vi "Set Tube State.vi"(4 "State":T1(ring), 5 "valve refs":refnum<vi>[](array[refnum]), 6 "error in":errorcluster, 8 "tube state ref":refnum<vi>, 9 "task in":refnum<k21>) -> (0 "error out":errorcluster, 3 "task out":refnum<k21>)   [LabVIEW 2018]
uses:
  <vilib>/DAQmx/write.llb/DAQmx Write (Digital 1D Bool 1Chan 1Samp).vi
  <vilib>/DAQmx/miscellaneous.llb/DAQmx Fill In Error Info.vi
panel:
  out "Valve Tube Inlet":bool caption="Tube Inlet"
  out "Valve Mix Inlet":bool caption="Mix Inlet"
  out "Valve Mix Outlet":bool caption="Mix Outlet"
  out "Valve Tube Outlet":bool=TRUE caption="Tube Outlet"
  out "Valve Oxidizer":bool caption="Oxidizer"
  out "Valve Fuel":bool caption="Fuel"
  out "Valve Diluent":bool caption="Diluent"
  out "Valve Purge":bool caption="Purge"
  out "Valve Vacuum":bool caption="Vacuum"
  out "Spark":bool
  out "Mix Fan":bool
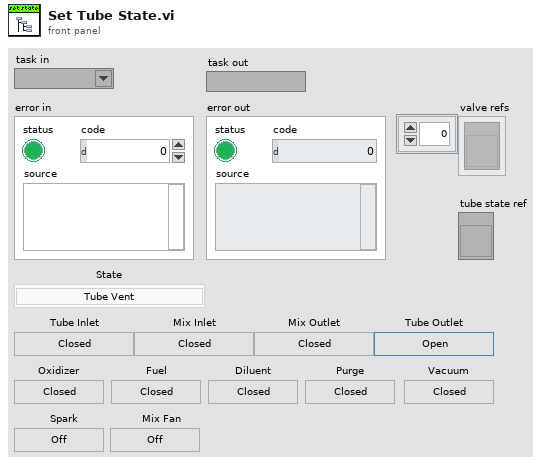
[diagram p1: front panel]
types:
  T1 = enum16{"Tube Vent", "Mix Section Purge", "Tube Purge", "Tube Vacuum", "Diluent Fill", "Oxidizer Fill", "Fuel Fill", "Fill Hold", "Mixing", "Tube Closed", "Ignition", "Manifold Vent"}
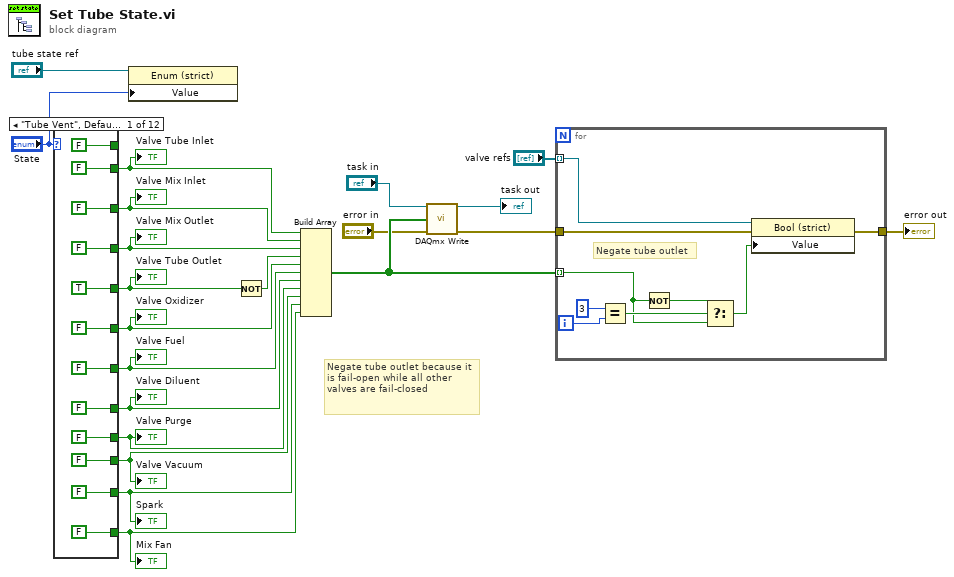
[diagram p0: block diagram]
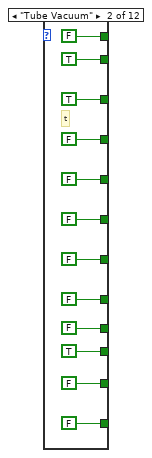
[diagram p2: hidden frame]
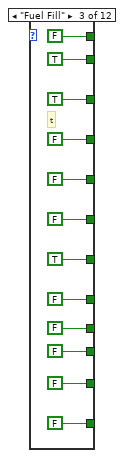
[diagram p3: hidden frame]
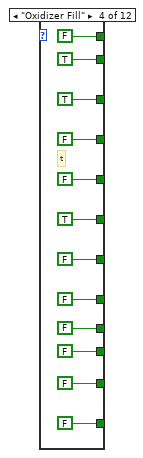
[diagram p4: hidden frame]
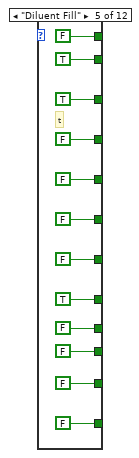
[diagram p5: hidden frame]
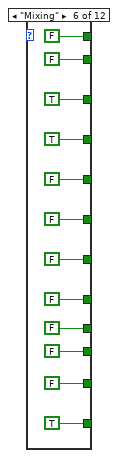
[diagram p6: hidden frame]
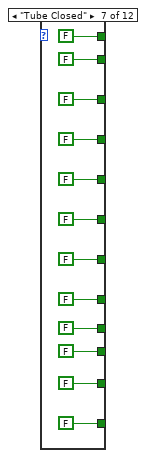
[diagram p7: hidden frame]
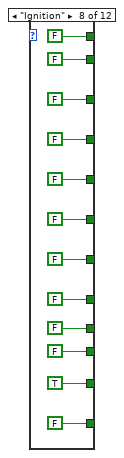
[diagram p8: hidden frame]
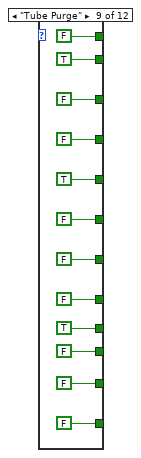
[diagram p9: hidden frame]
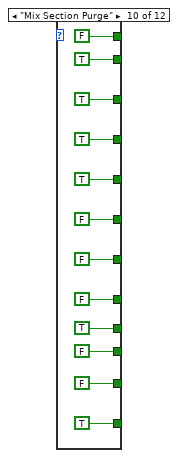
[diagram p10: hidden frame]
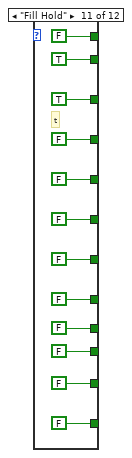
[diagram p11: hidden frame]
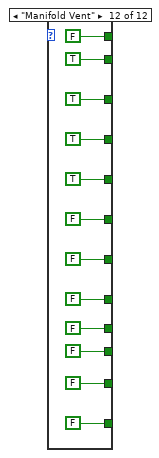
[diagram p12: hidden frame]
diagram:
  # "Negate tube outlet because it is fail-open while all other valves are fail-closed"
  n1 = case shown="\"Tube Vent\", Default" "State" {
    tunnel: [FALSE ("Vacuum") FALSE ("Vacuum") FALSE ("Vacuum") FALSE ("Vacuum") TRUE ("Vacuum") FALSE ("Vacuum") FALSE ("Vacuum") FALSE ("Vacuum") FALSE ("Vacuum") FALSE ("Vacuum") FALSE ("Vacuum") FALSE ("Vacuum")] -> w13
    tunnel: [FALSE ("Manifold Outlet") FALSE ("Manifold Outlet") TRUE ("Manifold Outlet") FALSE ("Manifold Outlet") FALSE ("Manifold Outlet") FALSE ("Manifold Outlet") FALSE ("Manifold Outlet") FALSE ("Manifold Outlet") FALSE ("Manifold Outlet") FALSE ("Manifold Outlet") FALSE ("Manifold Outlet") FALSE ("Manifold Outlet")] -> w14
    tunnel: [FALSE ("Purge") FALSE ("Purge") FALSE ("Purge") TRUE ("Purge") FALSE ("Purge") FALSE ("Purge") FALSE ("Purge") FALSE ("Purge") FALSE ("Purge") FALSE ("Purge") FALSE ("Purge") FALSE ("Purge")] -> w15
    tunnel: [FALSE ("Oxidizer") FALSE ("Oxidizer") FALSE ("Oxidizer") FALSE ("Oxidizer") FALSE ("Oxidizer") FALSE ("Oxidizer") FALSE ("Oxidizer") FALSE ("Oxidizer") TRUE ("Oxidizer") TRUE ("Oxidizer") FALSE ("Oxidizer") FALSE ("Oxidizer")] -> w12
    tunnel: [FALSE ("Fuel") TRUE ("Fuel") FALSE ("Fuel") FALSE ("Fuel") FALSE ("Fuel") FALSE ("Fuel") FALSE ("Fuel") FALSE ("Fuel") FALSE ("Fuel") FALSE ("Fuel") FALSE ("Fuel") FALSE ("Fuel")] -> w11
    tunnel: [FALSE ("Tube Inlet") TRUE ("Tube Inlet") TRUE ("Tube Inlet") TRUE ("Tube Inlet") TRUE ("Tube Inlet") FALSE ("Tube Inlet") FALSE ("Tube Inlet") FALSE ("Tube Inlet") TRUE ("Tube Inlet") TRUE ("Tube Inlet") TRUE ("Tube Inlet") TRUE ("Tube Inlet")] -> w19
    tunnel: [TRUE ("Tube Outlet") FALSE ("Tube Outlet") FALSE ("Tube Outlet") FALSE ("Tube Outlet") FALSE ("Tube Outlet") FALSE ("Tube Outlet") FALSE ("Tube Outlet") FALSE ("Tube Outlet") TRUE ("Tube Outlet") TRUE ("Tube Outlet") FALSE ("Tube Outlet") TRUE ("Tube Outlet")] -> w16
    tunnel: [FALSE ("Mix Inlet") TRUE ("Mix Inlet") TRUE ("Mix Inlet") TRUE ("Mix Inlet") TRUE ("Mix Inlet") TRUE ("Mix Inlet") FALSE ("Mix Inlet") FALSE ("Mix Inlet") FALSE ("Mix Inlet") TRUE ("Mix Inlet") TRUE ("Mix Inlet") TRUE ("Mix Inlet")] -> w18
    tunnel: [FALSE ("Mix Outlet") FALSE ("Mix Outlet") FALSE ("Mix Outlet") FALSE ("Mix Outlet") FALSE ("Mix Outlet") TRUE ("Mix Outlet") FALSE ("Mix Outlet") FALSE ("Mix Outlet") FALSE ("Mix Outlet") TRUE ("Mix Outlet") FALSE ("Mix Outlet") TRUE ("Mix Outlet")] -> w17
    tunnel: [FALSE ("Oxidizer") FALSE ("Vacuum") FALSE ("Purge") FALSE ("Oxidizer") FALSE ("Purge") FALSE ("Oxidizer") FALSE ("Oxidizer") TRUE ("Oxidizer") FALSE ("Vacuum") FALSE ("Vacuum") FALSE ("Oxidizer") FALSE ("Oxidizer")] -> w10
    tunnel: [FALSE ("Fuel") FALSE ("Manifold Outlet") FALSE ("Oxidizer") FALSE ("Fuel") FALSE ("Oxidizer") TRUE ("Fuel") FALSE ("Fuel") FALSE ("Fuel") FALSE ("Manifold Outlet") TRUE ("Manifold Outlet") FALSE ("Fuel") FALSE ("Fuel")] -> w9
    tunnel: [FALSE ("Diluent") FALSE ("Purge") FALSE ("Fuel") FALSE ("Diluent") FALSE ("Fuel") FALSE ("Diluent") FALSE ("Diluent") FALSE ("Diluent") FALSE ("Purge") FALSE ("Purge") FALSE ("Diluent") FALSE ("Diluent")] -> _
    frame "Tube Vent", Default {
    }
    frame "Tube Vacuum" {
      # "t"
    }
    frame "Fuel Fill" {
      # "t"
    }
    frame "Oxidizer Fill" {
      # "t"
    }
    frame "Diluent Fill" {
      # "t"
    }
    frame "Mixing" {
    }
    frame "Tube Closed" {
    }
    frame "Ignition" {
    }
    frame "Tube Purge" {
    }
    frame "Mix Section Purge" {
    }
    frame "Fill Hold" {
      # "t"
    }
    frame "Manifold Vent" {
    }
  }
  "Valve Tube Outlet" <- w16
  "Valve Mix Outlet" <- w17
  "Valve Mix Inlet" <- w18
  "Valve Tube Inlet" <- w19
  "Valve Purge" <- w12
  "Valve Diluent" <- w13
  "Valve Fuel" <- w14
  "Valve Oxidizer" <- w15
  "Valve Vacuum" <- w11
  "Spark" <- w10
  "Mix Fan" <- w9
  n2 = property class="Enum (strict)"(reference="tube state ref", "Value"="State") -> ()  [unwired: 1 in, 2 out]
  n3 = Not(x=w16) -> (.not. x?=w3:bool)
  n4 = Build Array(w19, w18, w17, w3, w15, w14, w13, w12, w11, w10, w9) -> (w7:bool[])
  n5 = call-poly <vilib>:"DAQmx Write.vi"("task/channels in"="task in", "data"=w7, "error in"="error in") -> ("task out"=→"task out":refnum<k21>, "error out"=w4:errorcluster)  [unwired: 10 in, 1 out]
  n6 = for {
    tunnel: "valve refs" -> [w174] mode=indexing
    tunnel: w7 -> [w167] mode=indexing
    tunnel: [w173] -> w20
    tunnel: w4 -> [w172]
    i -> [w171]
    # "Negate tube outlet"
    n7 = Equal?(x=3, y=w171) -> (x = y?=w169:bool)
    n8 = Not(x=w167) -> (.not. x?=w168:bool)
    n9 = Select(t=w168, s=w169, f=w167) -> (s? t:f=w166:bool)
    n10 = property class="Bool (strict)"(reference=w174, error in=w172, "Value"=w166) -> (error out=w173:errorcluster)  [unwired: 1 out]
  }
  "error out" <- w20
